vi "Confirure FIFO Depths (SubVI).vi"(8 "error in (no error)":errorcluster, 11 "Refnum in":refnum<k20>) -> (0 "error out":errorcluster, 1 "Actual Depth 3":u32, 2 "Actual Depth 2":u32, 3 "Refnum out":refnum<k20>, 4 "Actual Depth 4":u32, 5 "Actual Depth":u32)   [LabVIEW 2017]
uses:
  <vilib>/Utility/error.llb/Error Cluster From Error Code.vi
  <vilib>/rvi/interface/common/niFpgaWaitOnOcc.vi
  <vilib>/rvi/interface/nirviMethod/nirviMethod.xnode
  <vilib>/FPGAPlugInAG/Dynamic/niLvFpga_ConfigureFifo_Dynamic.vi
  <vilib>/rvi/errors/niLvFpgaMergeErrorWithErrorCode.vi
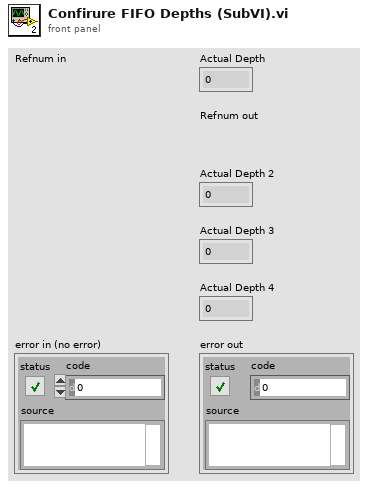
[diagram p1: front panel]
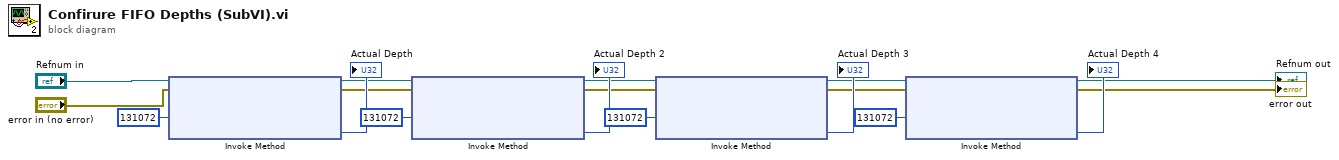
[diagram p0: block diagram]
diagram:
  n1 = xnode "Invoke Method"("FPGA VI Reference In"="Refnum in", "error in"="error in (no error)", "Requested Depth"=u32 131072) -> ("FPGA VI Reference Out"=w7:refnum<k20>, "error out"=w11:errorcluster, "Actual Depth"=→"Actual Depth":u32)
  n2 = xnode "Invoke Method"("FPGA VI Reference In"=w7, "error in"=w11, "Requested Depth"=u32 131072) -> ("FPGA VI Reference Out"=w8:refnum<k20>, "error out"=w12:errorcluster, "Actual Depth"=→"Actual Depth 2":u32)
  n3 = xnode "Invoke Method"("FPGA VI Reference In"=w8, "error in"=w12, "Requested Depth"=u32 131072) -> ("FPGA VI Reference Out"=w9:refnum<k20>, "error out"=w13:errorcluster, "Actual Depth"=→"Actual Depth 3":u32)
  n4 = xnode "Invoke Method"("FPGA VI Reference In"=w9, "error in"=w13, "Requested Depth"=u32 131072) -> ("FPGA VI Reference Out"=→"Refnum out":refnum<k20>, "error out"=→"error out":errorcluster, "Actual Depth"=→"Actual Depth 4":u32)
